vi "Screen Saver Control.vi"(8 "error in (no error)":errorcluster, 10 "screen saver settings (60s, T)":cluster{"timeout value":u32, "active?":bool}={"timeout value"=60, "active?"=TRUE} {"timeout value" min=1}, 11 "function (0:Get Info)":T1(ring)) -> (0 "error out":errorcluster, 2 "screen saver settings":cluster{"timeout value":u32, "active?":bool})   [LabVIEW 2020, in "MacroAssert.lvlib" / "Winsys.lvlib"]
doc: "This VI provides the user with the ability to get or set the timeout of the screensaver, as well as determine whether the screen saver is active."
uses:
  Winsys.lvlib
  user32.dll
  kernel32.dll
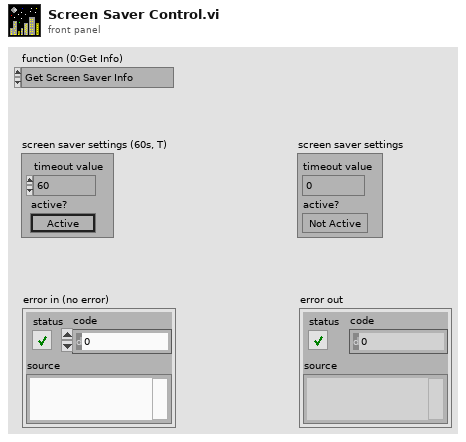
[diagram p1: front panel]
types:
  T1 = enum8{"Get Screen Saver Info", "Set Screen Saver Info"}
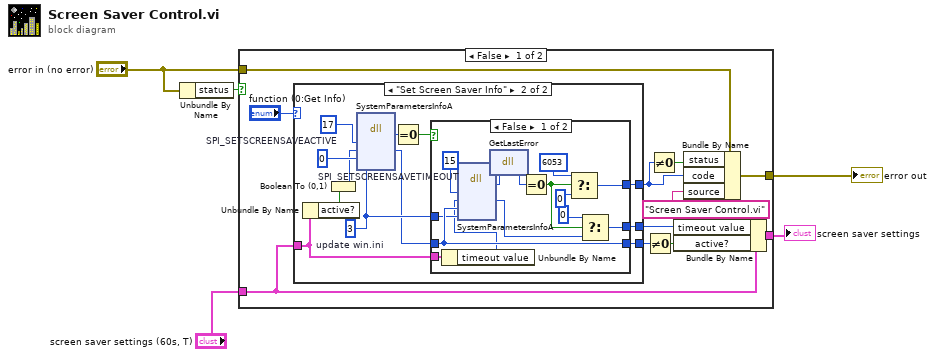
[diagram p0: block diagram]
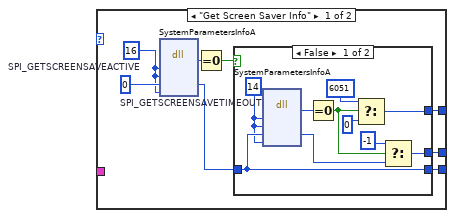
[diagram p2: hidden frame]
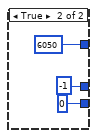
[diagram p3: hidden frame]
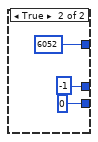
[diagram p4: hidden frame]
diagram:
  n1 = Unbundle By Name("error in (no error)") -> ("status"=w3:bool)
  n2 = case shown="False" w3 {
    tunnel: "screen saver settings (60s, T)" -> [w6 w67]
    tunnel: "error in (no error)" -> [w7 w68]
    tunnel: [w9 w68] -> w1
    tunnel: [w8 w67] -> w4
    frame False {
      n3 = case shown="\"Set Screen Saver Info\"" "function (0:Get Info)" {
        tunnel: [w19 w46] -> w11
        tunnel: [w18 w45] -> w13
        tunnel: [w17 w44] -> w15
        tunnel: w6 -> [_ w39]
        frame "Get Screen Saver Info" {
          w20 = u32 16  # SPI_GETSCREENSAVEACTIVE
          n4 = dll-call lib="user32.dll" fn="SystemParametersInfoA"(w20, w20, 0, w20) -> (w23:i32, w21:i32)  [unwired: 6 in, 2 out]
          n5 = Equal To 0?(x=w23) -> (x = 0?=w22:bool)
          n6 = case shown="False" w22 {
            tunnel: w21 -> [w26 _]
            tunnel: [w28 i16 -1] -> w18
            tunnel: [w27 6050] -> w19
            tunnel: [w26 i16 0] -> w17
            frame False {
              w25 = u32 14  # SPI_GETSCREENSAVETIMEOUT
              n7 = dll-call lib="user32.dll" fn="SystemParametersInfoA"(w25, w25, w26, w25) -> (w34:i32, w29:i32)  [unwired: 6 in, 2 out]
              n8 = Equal To 0?(x=w34) -> (x = 0?=w31:bool)
              n9 = Select(t=6051, s=w31, f=0) -> (s? t:f=w27:i32)
              n10 = Select(t=i16 -1, s=w31, f=w29) -> (s? t:f=w28:i32)
            }
            frame True {
            }
          }
        }
        frame "Set Screen Saver Info" {
          w43 = u32 3  # update win.ini
          w42 = u32 17  # SPI_SETSCREENSAVEACTIVE
          n11 = Unbundle By Name(w39) -> ("active?"=w41:bool)
          n12 = Boolean To (0,1)(Boolean=w41) -> (0, 1=w40:i16)
          n13 = dll-call lib="USER32.DLL" fn="SystemParametersInfoA"(w42, w40, 0, w43) -> (w48:i32, w38:u32)  [unwired: 6 in, 2 out]
          n14 = Equal To 0?(x=w48) -> (x = 0?=w47:bool)
          n15 = case shown="False" w47 {
            tunnel: w38 -> [w57 _]
            tunnel: [w59 i16 -1] -> w45
            tunnel: [w58 6052] -> w46
            tunnel: [w57 i16 0] -> w44
            tunnel: w43 -> [w56 _]
            tunnel: w39 -> [w54 _]
            frame False {
              w55 = u32 15  # SPI_SETSCREENSAVETIMEOUT
              n16 = Unbundle By Name(w54) -> ("timeout value"=w53:u32)
              n17 = dll-call lib="USER32.DLL" fn="SystemParametersInfoA"(w55, w53, w57, w56) -> (w51:i32, w52:u32)  [unwired: 6 in, 2 out]
              n18 = dll-call lib="kernel32.dll" fn="GetLastError"(w51) -> (w50:i32)  [unwired: 2 in, 2 out]
              n19 = Equal To 0?(x=w50) -> (x = 0?=w61:bool)
              n20 = Select(t=6053, s=w61, f=0) -> (s? t:f=w58:i32)
              n21 = Select(t=u16 0, s=w61, f=w52) -> (s? t:f=w59:u32)
            }
            frame True {
            }
          }
        }
      }
      n22 = Not Equal To 0?(x=w15) -> (x != 0?=w14:bool)
      n23 = Not Equal To 0?(x=w11) -> (x != 0?=w12:bool)
      n24 = Bundle By Name(cluster=w6, "timeout value"=w13, "active?"=w14) -> (w8:cluster{"timeout value":u32, "active?":bool})
      n25 = Bundle By Name(cluster=w7, "status"=w12, "code"=w11, "source"="Screen Saver Control.vi") -> (w9:errorcluster)
    }
    frame True {
    }
  }
  "screen saver settings" <- w4
  "error out" <- w1
